vi "Validate Instrument Addon Refnum.vi"(8 "Error In":errorcluster, 11 "Refnum In":T1 format="%.0x") -> (0 "Error Out":errorcluster, 2 "Is Instrument Addon?":bool, 3 "Refnum Out":T1 format="%.0x")   [LabVIEW 2018, in "Instrument Addon Scripting API.lvlib"]
doc: "Verifies if the provided Refnum is an Instrument Addon Custom Device\n\nInput: \nRefnum In: represent the reference number which about to be compared agains the Instrument Addon GUID\n\nOutput: \nRefnum Out: represents the reference number provided as input\nIs Instrument Addon?: boolean value which indicates if the provided refnum references an Instrument Addon Custom Device"
uses:
  Instrument Addon Scripting API.lvlib
  <vilib>/NI Veristand/Custom Device API/Custom Device Item Ref.ctl
  Addon/Addon Shared/SubVIs/Constants.vi
  <vilib>/NI/NI VeriStand Advanced SysDef API/SysDef API/Advanced System Definition.lvlib
  Addon/Addon Shared/Instrument Addon Shared.lvlib
  <vilib>/NI Veristand/Custom Device API/Custom Device API.lvlib
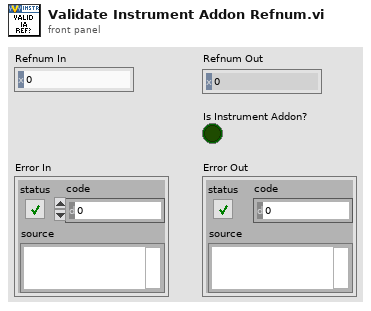
[diagram p1: front panel]
types:
  T1 = typedef "Custom Device API.lvlib/Custom Device Item Ref.ctl" = u64
  T2 = typedef "Advanced System Definition.lvlib/TreeItem.Info.ctl" = cluster{"Name":string, "Description":string, "GUID":string, "Is Channel":bool, "Channel":T3, "Is Waveform":bool, "Waveform":T5}
  T3 = typedef "Custom Device API.lvlib/Custom Device Channel.ctl" = cluster{"Type":T4, "Units":string, "Default Value":dbl, "Faultable":bool, "Scalable":bool}
  T4 = typedef "Custom Device API.lvlib/Custom Device Channel Type.ctl" = enum16{"Input", "Output"}
  T5 = typedef "Custom Device API.lvlib/Custom Device Waveform.ctl" = cluster{"Data Type":T6, "Units":string}
  T6 = typedef "Custom Device API.lvlib/Custom Device Waveform DataType.ctl" = enum16{"Double", "Complex Double"}
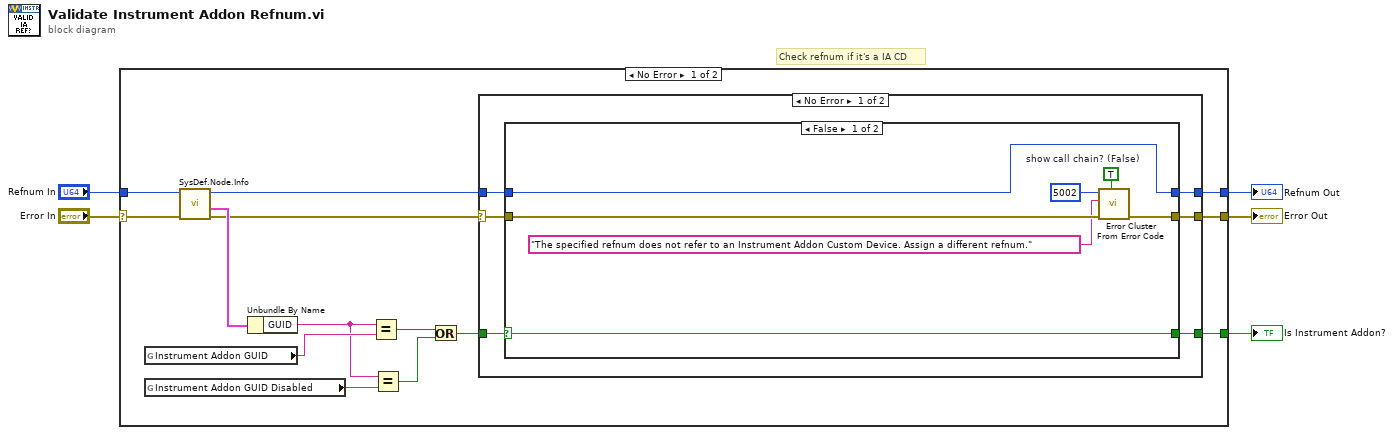
[diagram p0: block diagram]
diagram:
  # "Check refnum if it's a IA CD"
  n1 = case shown="No Error" "Error In" {
    selector: "Error In" -> [w16 w39]
    tunnel: [w15 w39] -> w5
    tunnel: [w13 w40] -> w1
    tunnel: "Refnum In" -> [w17 w40]
    tunnel: [w12 _] -> w3
    frame No Error {
      n2 = global read "Constants.vi" "Instrument Addon GUID"() -> (w19:string)
      n3 = global read "Constants.vi" "Instrument Addon GUID Disabled"() -> (w10:string)
      n4 = call <vilib>:"SysDef.Node.Info.vi"("error in (no error)"=w16, "nodeID"=w17) -> ("error out"=w11:errorcluster, "Item Info"=w18:T2, "nodeID out"=w14:u64)  [unwired: 6 in, 1 out]
      n5 = Unbundle By Name(w18) -> ("GUID"=w9:string)
      n6 = Equal?(x=w9, y=w19) -> (x = y?=w6:bool)
      n7 = Equal?(x=w9, y=w10) -> (x = y?=w8:bool)
      n8 = Or(x=w6, y=w8) -> (x .or. y?=w7:bool)
      n9 = case shown="No Error" w11 {
        selector: w11 -> [w21 w38]
        tunnel: [w25 w38] -> w15
        tunnel: w14 -> [w24 w37]
        tunnel: [w23 w37] -> w13
        tunnel: [w22 w36] -> w12
        tunnel: w7 -> [w20 w36]
        frame No Error {
          n10 = case shown="False" w20 {
            selector: w20 -> [w31 w34]
            tunnel: [w30 w33] -> w25
            tunnel: w24 -> [w32 w35]
            tunnel: [w32 w35] -> w23
            tunnel: [w31 w34] -> w22
            tunnel: w21 -> [w29 w33]
            frame False {
              w26 = TRUE  # show call chain? (False)
              n11 = call <vilib>:"Error Cluster From Error Code.vi"("show call chain? (False)"=w26, "error in (no error)"=w29, "error message (\"\")"="The specified refnum does not refer to an Instrument Addon Custom Device. Assign a different refnum." ("error message (\"\")"), "error code (0)"=5002) -> ("error out"=w30:errorcluster)  [unwired: 5 in]
            }
            frame True {
            }
          }
        }
        frame Error {
        }
      }
    }
    frame Error {
    }
  }
  "Error Out" <- w5
  "Is Instrument Addon?" <- w3
  "Refnum Out" <- w1
